vi "SP Build Query - DataFinder.vi"(8 "error in (no error)":errorcluster, 10 "UserName":string, 11 "Fields":T2[](array[typedef])) -> (0 "error out":errorcluster, 3 "Field Information":T1[](array[typedef]))   [LabVIEW 2011]
uses:
  server/DIAdem/lib/DIAdem Query Data.ctl
  server/DataFinder/DataFinder Comparisons.ctl
  cgi-bin/_cgi-lib/TDM_INDEX Record.ctl
  server/DataFinder/Datafinder Query.ctl
  server/DataFinder/eSearch Types.ctl
  server/DIAdem/Datasheet/Query Parameters.ctl
  server/DIAdem/lib/DIAdem Query Queue.ctl
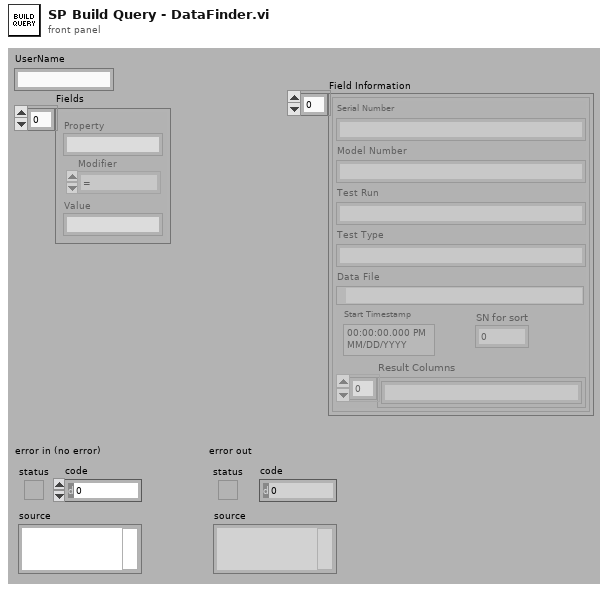
[diagram p1: front panel]
types:
  T1 = typedef "TDM_INDEX Record.ctl" = cluster{"Model Number":string, "SN for sort":i32, "Test Type":string, "Test Run":string, "Serial Number":string, "Start Timestamp":timestamp, "Data File":path, "Result Columns":string[]}
  T2 = typedef "DIAdem Query Data.ctl" = cluster{"Property":string, "Modifier":T3, "Value":string}
  T3 = typedef "DataFinder Comparisons.ctl" = enum16{"=", "<>", "<", "<=", ">", ">="}
  T4 = typedef "DIAdem Query Queue.ctl" = cluster{"UserName":string, "Search Parameters":T5[], "eSearch Type":T6, "Query Name (vbs)":string, "Response queue name":string, "Logic String":string}
  T5 = typedef "Datafinder Query.ctl" = cluster{"eSearch Types":T6, "Property Name":string, "DataFinder Comparisons":T3, "Property Value":string}
  T6 = typedef "eSearch Types.ctl" = enum16{"eSearchFile", "eSearchChannelGroup", "eSearchChannel"}
  T7 = typedef "Query Parameters.ctl" = cluster{"Action":string, "Serial Number":string, "Model Number":string, "MNWILD":string, "StartDate":string, "EndDate":string, "DateCOMP":string, "Conditions":T5[], "MN Wild List":string[], "SN by MN Wild List":cluster{"Serial Number List":string[]}[], "Recall Table?":bool, "Type":string, "Show Date?":bool, "Show Conditions?":bool, "Serial Number Display Name":string, "Model Number Display Name":string, "Test Type String":string, "Manager":bool, "Custom Rows":string[][], "Custom Result HTML":string, "User Name":string, "State":string, "MN Query ":string, "SN Query":string, "Custom Analysis HTML":string, "RUNSELECT":string}
  T8 = typedef "Connection Refnum.ctl" = cluster{"Environment Handle":i32, "Connection Handle":i32}
  T9 = typedef "DIAdem Query Result.ctl" = cluster{"Results":string[][], "# of Items":i32, "Data Returned?":bool, "Result TDM":path, "Timed Out?":bool}
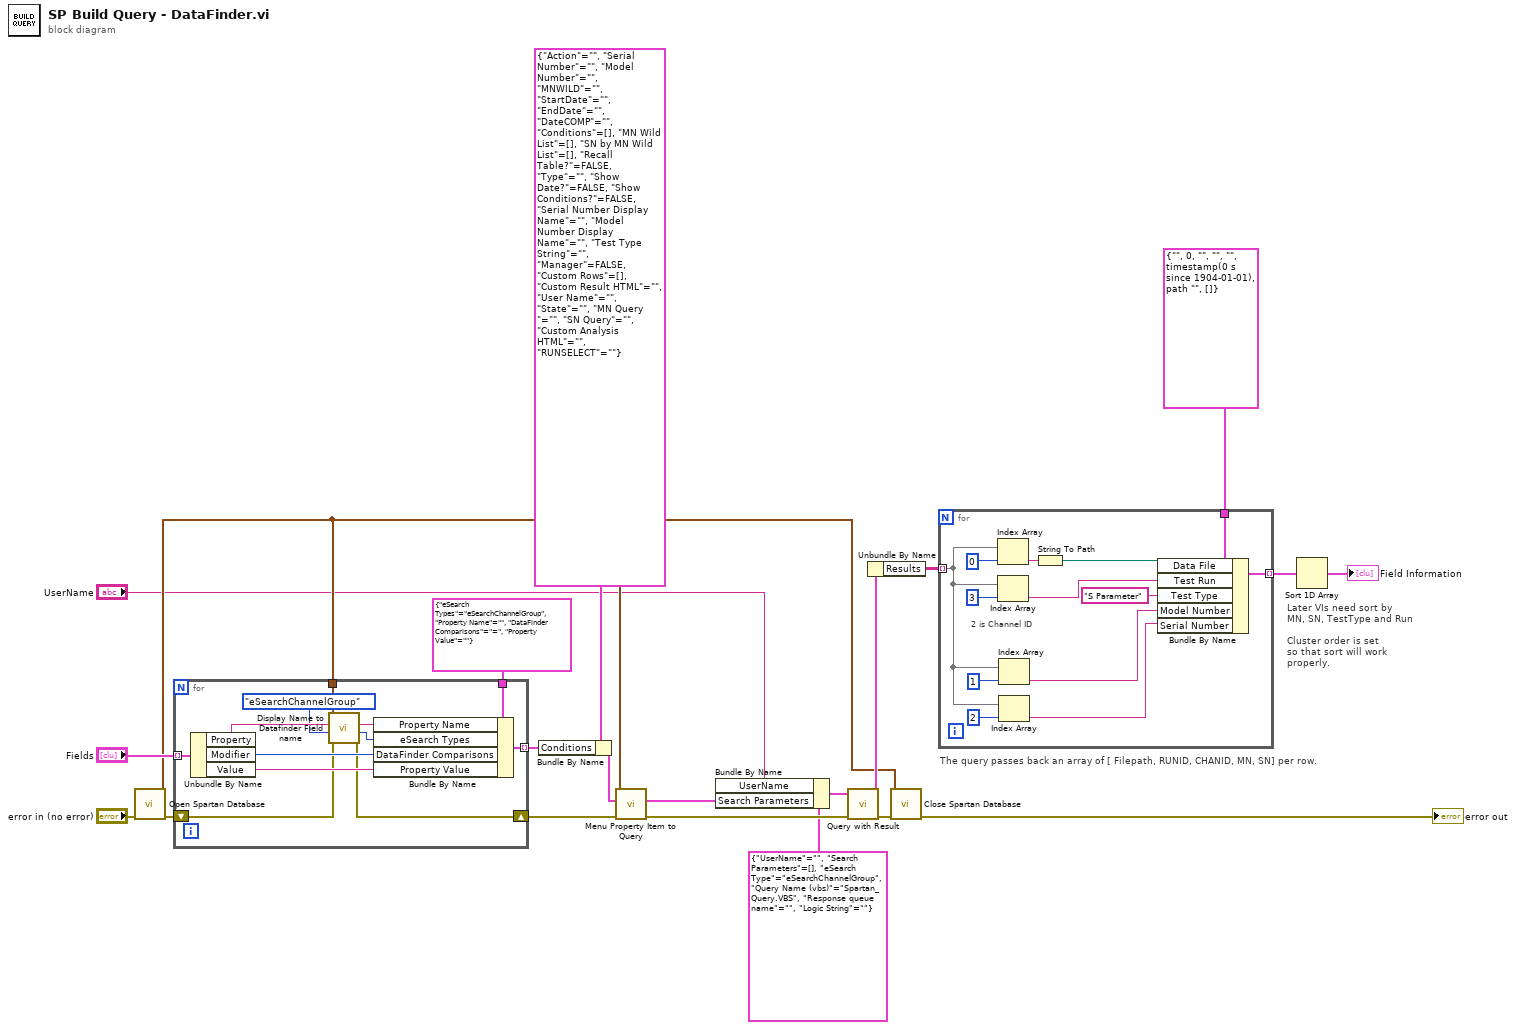
[diagram p0: block diagram]
diagram:
  # "The query passes back an array of [ Filepath, RUNID, CHANID, MN, SN] per row."
  # "Later VIs need sort by \nMN, SN, TestType and Run\n\nCluster order is set\nso that sort will work\nproperly."
  n1 = call "Open Spartan Database.vi"("error in (no error)"="error in (no error)") -> ("error out"=w7:errorcluster, "Connection Refnum"=w8:T8)  [unwired: 1 in, 8 out]
  n2 = for {
    tunnel: "Fields" -> [w33] mode=indexing
    tunnel: [w30] -> w14 mode=indexing
    tunnel: T5 {"eSearch Types"=enum."eSearchChannelGroup", "Property Name"="", "DataFinder Comparisons"=enum."=", "Property Value"=""} ("Data Finder Parameters") -> [w29]
    tunnel: w8 -> [w24]
    shift-right: [w22] -> w6
    shift-left: w7 -> [w23]
    n3 = Unbundle By Name(w33) -> ("Property"=w28:string, "Modifier"=w32:T3, "Value"=w31:string)
    n4 = call "Display Name to Datafinder Field name.vi"("error in (no error)"=w23, "eSearch Type In"=eSearch_Types."eSearchChannelGroup" ("eSearch Types"), "Field Display Name"=w28, "Connection Refnum"=w24) -> ("error out"=w22:errorcluster, "eSearch Type Out"=w25:T6, "Datafinder Search Name"=w26:string)  [unwired: 5 out]
    n5 = Bundle By Name(cluster=w29, "Property Name"=w26, "eSearch Types"=w25, "DataFinder Comparisons"=w32, "Property Value"=w31) -> (w30:T5)
  }
  n6 = Bundle By Name(cluster=T7 {"Action"="", "Serial Number"="", "Model Number"="", "MNWILD"="", "StartDate"="", "EndDate"="", "DateCOMP"="", "Conditions"=[], "MN Wild List"=[], "SN by MN Wild List"=[], "Recall Table?"=FALSE, "Type"="", "Show Date?"=FALSE, "Show Conditions?"=FALSE, "Serial Number Display Name"="", "Model Number Display Name"="", "Test Type String"="", "Manager"=FALSE, "Custom Rows"=[], "Custom Result HTML"="", "User Name"="", "State"="", "MN Query "="", "SN Query"="", "Custom Analysis HTML"="", "RUNSELECT"=""} ("Custom Search Parameters"), "Conditions"=w14) -> (w13:T7)
  n7 = call "Menu Property Item to Query.vi"("error in (no error)"=w6, "Custom Search Parameters"=w13, "Connection Refnum In"=w8) -> ("error out"=w12:errorcluster, "Custom Search Parameters"=w1:T5[])  [unwired: 7 out]
  n8 = Bundle By Name(cluster=T4 {"UserName"="", "Search Parameters"=[], "eSearch Type"=enum."eSearchChannelGroup", "Query Name (vbs)"="Spartan_Query.VBS", "Response queue name"="", "Logic String"=""} ("Query Parameter Data"), "UserName"="UserName", "Search Parameters"=w1) -> (w3:T4)
  n9 = call "Query with Result.vi"("error in (no error)"=w12, "Query Parameter Data"=w3) -> ("error out"=w10:errorcluster, "Query Return Data"=w20:T9)  [unwired: 1 in, 7 out]
  n10 = Unbundle By Name(w20) -> ("Results"=w5:string[][])
  n11 = call "Close Spartan Database.vi"("error in (no error)"=w10, "Connection Refnum"=w8) -> ("error out"=→"error out":errorcluster)  [unwired: 2 in, 7 out]
  n12 = for {
    tunnel: w5 -> [w38] mode=indexing
    tunnel: T1 {"Model Number"="", "SN for sort"=0, "Test Type"="", "Test Run"="", "Serial Number"="", "Start Timestamp"=timestamp(0 s since 1904-01-01), "Data File"=path "", "Result Columns"=[]} ("Station Information") -> [w46]
    tunnel: [w41] -> w18 mode=indexing
    # "2 is Channel ID"
    n13 = Index Array(array=w38, index=0) -> (element=w43:string)
    n14 = Index Array(array=w38, index=3) -> (element=w42:string)
    n15 = Index Array(array=w38, index=1) -> (element=w37:string)
    n16 = Index Array(array=w38, index=2) -> (element=w36:string)
    n17 = String To Path(string=w43) -> (path=w35:path)
    n18 = Bundle By Name(cluster=w46, "Data File"=w35, "Test Run"=w42, "Test Type"="S Parameter", "Model Number"=w37, "Serial Number"=w36) -> (w41:T1)
  }
  n19 = Sort 1D Array(array=w18) -> (sorted array=→"Field Information":T1[])
